vi "Teleop.vi"(10 "Match Info":T2={"Autonomous Elapsed Seconds"=0.0, "TeleOp Elapsed Seconds"=0.0, "Disabled Elapsed Seconds"=0.0, "Visited Autonomous"=FALSE, "Visited TeleOp"=FALSE, "Visited Disabled"=FALSE, "Autonomous Settings"={"Autonomous Style"=enum."Independent", "VI Refnum"=refnum}}, 11 "Call Context":T3) -> ()   [LabVIEW 2020]
doc: "This VI is called for each TeleOp packet received from the DS where the robot is not disabled. It is often used to read from the joysticks and update I/O or to update setpoints for timed control loops. It should complete and return within 20 milliseconds or it may miss DS packets."
uses:
  <vilib>/Rock Robotics/WPI/DriverStation/WPI_DriverStationDerivedRobotMode.ctl
  <vilib>/Rock Robotics/WPI/DriverStation/WPI_DriverStationMatch Info.ctl
  <vilib>/Rock Robotics/WPI/ThirdParty/Phoenix-LabVIEW/Motor Controller/Controls/CTRE_Phoenix_MotorControl_ControlMode.ctl
  <vilib>/Rock Robotics/WPI/Solenoid/WPI_SolenoidValue.ctl
  <vilib>/Rock Robotics/WPI/Utilities/WPI_GetSetVariantRefNum.vi
  <vilib>/Rock Robotics/Network Tables/NT Read Boolean.vi
  <vilib>/Rock Robotics/Network Tables/NT Read Number.vi
  <vilib>/Rock Robotics/Network Tables/NT Read String.vi
  <vilib>/Rock Robotics/Network Tables/NT Write Boolean.vi
  <vilib>/Rock Robotics/Network Tables/NT Write String.vi
  <vilib>/Rock Robotics/WPI/Solenoid/WPI_SolenoidSetEnum.vi
  <vilib>/Rock Robotics/WPI/ThirdParty/Phoenix-LabVIEW/Motor Controller/Get/CTRE_Phoenix_MotorController_IntegratedSensorData_TalonFX.vi
  <vilib>/Rock Robotics/Network Tables/NT Write Number.vi
  <vilib>/addons/control/pid/pid.llb/PID (DBL).vi
  <vilib>/addons/control/pid/NI_PID_pid.lvlib
panel:
  in  "PID gains 5":T1={"proportional gain (Kc)"=0.005, "integral time (Ti, min)"=0.0, "derivative time (Td, min)"=2e-05} {"derivative time (Td, min)" format="%.6f"; "integral time (Ti, min)" format="%.3f"; "proportional gain (Kc)" format="%.3f"}
  in  "Elevate want":dbl=-0.35
  in  "Intake want":dbl=0.75
  in  "Subtract rpm":dbl=2975.0
  out "% voltage":dbl
  out "voltage (V)":dbl
  out "Motor Volts":dbl
  out "rpm":dbl
  out "limelight tx":dbl
  out "limelight ty":dbl
  in  "Auto-Accept":bool
  in  "8togglePressed?":bool
  in  "Red/Blue":u32(colorbox)
  out "B":u8
  out "G":u8
  out "R":u8
  out "Color":u32(colorbox)
  out "Sample Slider 0":dbl(slide) scale=0.0..5.0
  out "Sample Boolean 1":bool
  out "Sample Boolean 0":bool
  # "-1"
  # "0"
  # ".75"
  # ".75"
  # "-.6"
  # "-.35"
  # ".1"
  # "1"
  # "-.1"
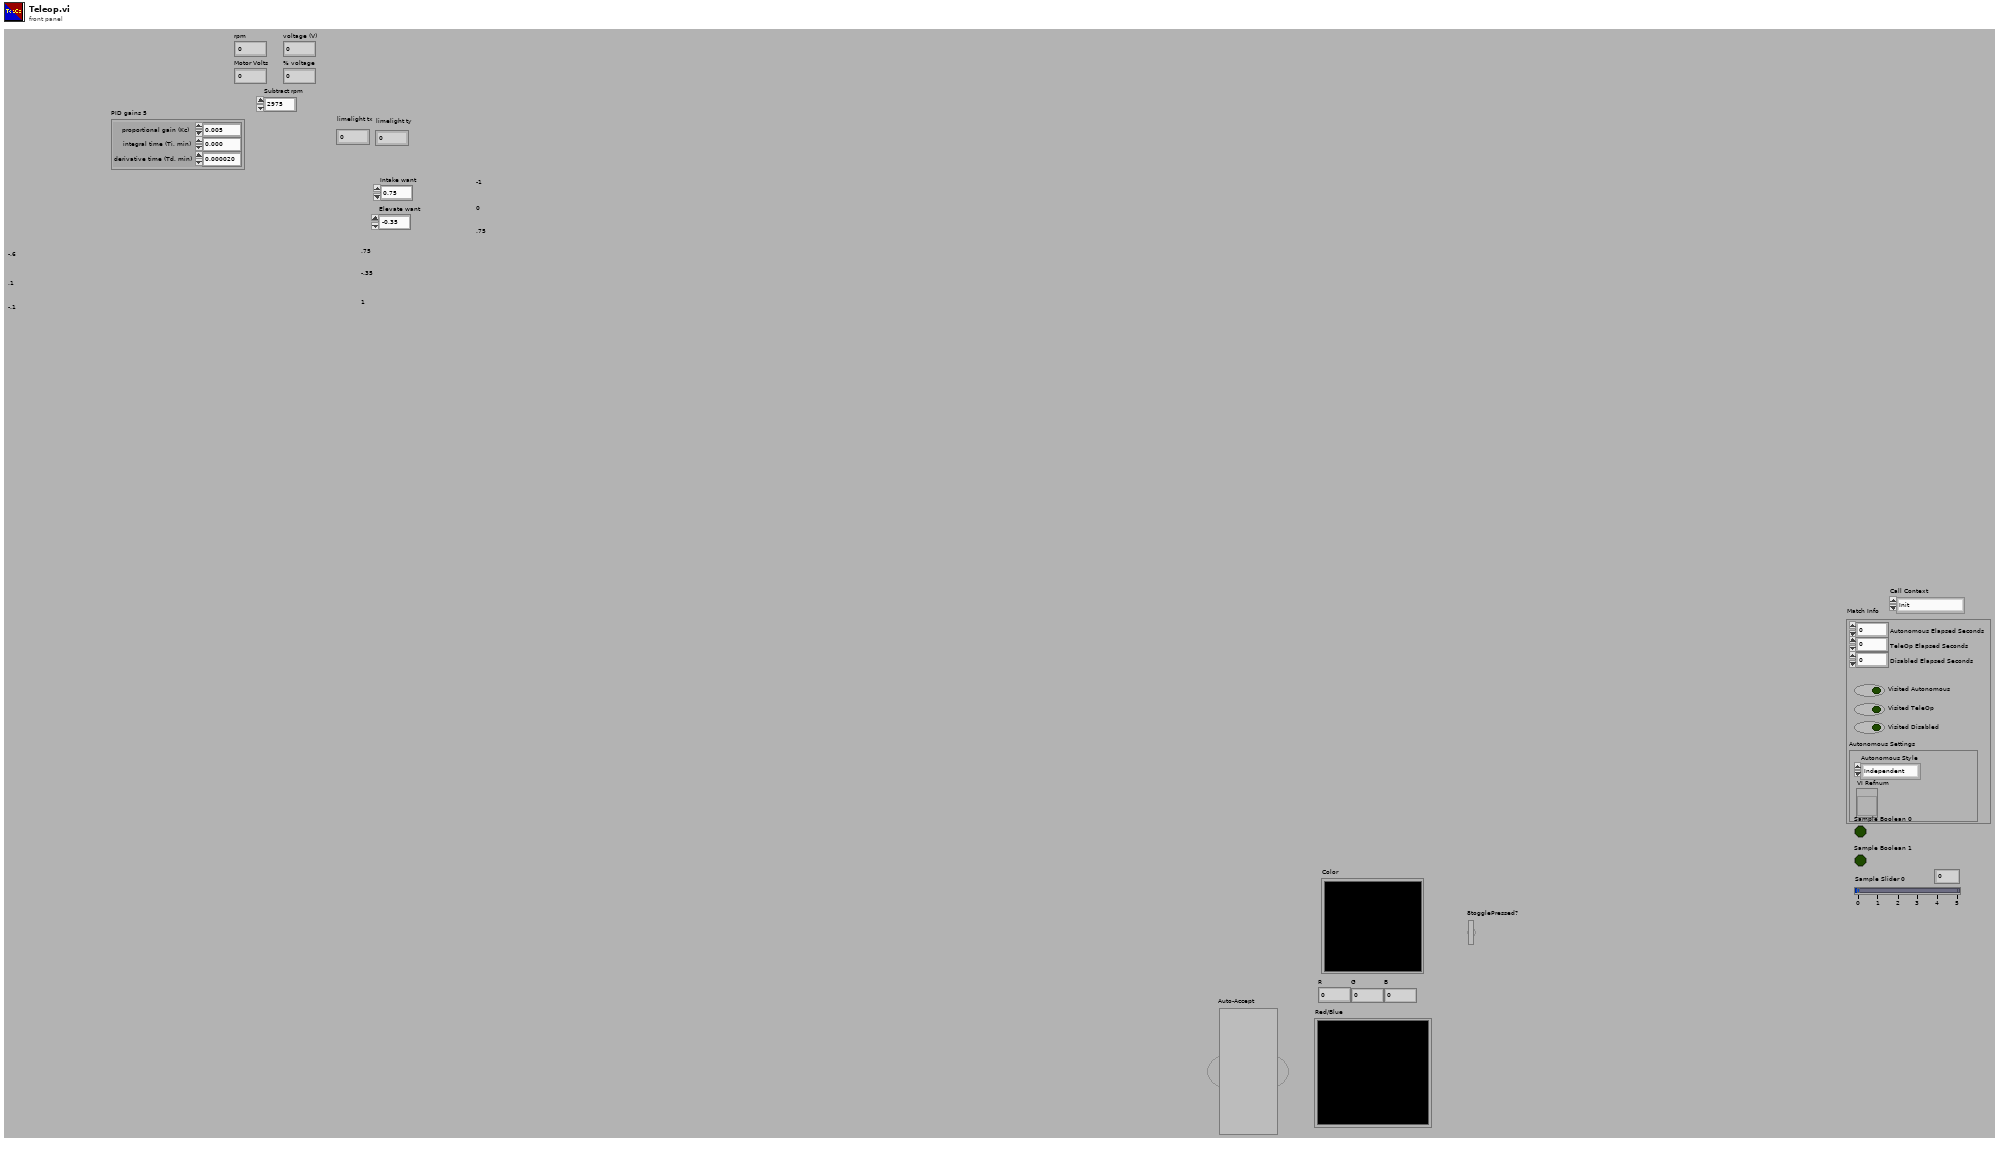
[diagram p1: front panel]
types:
  T1 = cluster{"proportional gain (Kc)":dbl, "integral time (Ti, min)":dbl, "derivative time (Td, min)":dbl}
  T2 = typedef "WPI_DriverStationMatch Info.ctl" = cluster{"Autonomous Elapsed Seconds":dbl, "TeleOp Elapsed Seconds":dbl, "Disabled Elapsed Seconds":dbl, "Visited Autonomous":bool, "Visited TeleOp":bool, "Visited Disabled":bool, "Autonomous Settings":cluster{"Autonomous Style":enum16{"Iterative", "Independent"}, "VI Refnum":refnum<vi>}}
  T3 = typedef "WPI_DriverStationDerivedRobotMode.ctl" = enum16{"Init", "Execute", "Stop"}
  T4 = typedef "CTRE_Phoenix_MotorControl_ControlMode.ctl" = u16
  T5 = typedef "WPI_SolenoidValue.ctl" = enum16{"Off", "On", "Forward", "Reverse"}
  T6 = typedef "WPI_MotorControlDeviceRef.ctl" = cluster{"DeviceStatus":errorcluster, "Type":T7, "PWM":cluster{"PWM Channel":T8, "DeadBand":T9}, "CAN":cluster{"Device Number":u8, "SetOutput VI Ref":variant, "GetOutput VI Ref":variant, "Enable VI Ref":variant, "Disable VI Ref":variant, "Data":variant}, "Invert":bool, "DIO PWM":cluster{"PWM \"Enable\" Channel":T8, "DIOChannel":T10, "PWM Rate":dbl}}
  T7 = typedef "WPI_MotorControlType.ctl" = enum16{"PWM", "CAN", "DIO PWM"}
  T8 = typedef "FPGA_DIOPWMChannel.ctl" = enum8{"PWM 0", "PWM 1", "PWM 2", "PWM 3", "PWM 4", "PWM 5", "PWM 6", "PWM 7", "PWM 8", "PWM 9", "PWM MXP 0", "PWM MXP 1", "PWM MXP 2", "PWM MXP 3", "PWM MXP 4", "PWM MXP 5", "PWM MXP 6", "PWM MXP 7", "PWM MXP 8", "PWM MXP 9", "Invalid"}
  T9 = typedef "WPI_PWMDeadband.ctl" = cluster{"Name":string, "maxPositivePwm":i32, "minPositivePwm":i32, "centerPwm":i32, "maxNegativePwm":i32, "minNegativePwm":i32, "angularRange":u16}
  T10 = typedef "FPGA_DIOChannel.ctl" = enum8{"DIO 0", "DIO 1", "DIO 2", "DIO 3", "DIO 4", "DIO 5", "DIO 6", "DIO 7", "DIO 8", "DIO 9", "DIO MXP 0", "DIO MXP 1", "DIO MXP 2", "DIO MXP 3", "DIO MXP 4", "DIO MXP 5", "DIO MXP 6", "DIO MXP 7", "DIO MXP 8", "DIO MXP 9", "DIO MXP 10", "DIO MXP 11", "DIO MXP 12", "DIO MXP 13", "DIO MXP 14", "DIO MXP 15", "SPI Port CS1", "SPI Port CS2", "SPI Port CS3", "SPI Port MISO", "SPI Port MOSI", "Invalid"}
  T11 = typedef "WPI_SolenoidDevRef.ctl" = cluster{"DevStatus":errorcluster, "Pneumatics Control Module":u8, "Forward Solenoid Channel":T12, "Reverse Solenoid Channel":T12}
  T12 = typedef "WPI_SolenoidChannel.ctl" = enum8{"Solenoid 0", "Solenoid 1", "Solenoid 2", "Solenoid 3", "Solenoid 4", "Solenoid 5", "Solenoid 6", "Solenoid 7", "Solenoid 8", "Solenoid 9", "Solenoid 10", "Solenoid 11", "Solenoid 12", "Solenoid 13", "Solenoid 14", "Solenoid 15", "Invalid"}
  T13 = typedef "WPI_CompressorDevRef.ctl" = cluster{"DevStatus":errorcluster, "Pneumatics Control Module":u8}
  T14 = typedef "WPI_SwitchDevRef.ctl" = cluster{"DevStatus":errorcluster, "DIO Channel":T10, "CntIndex":T15, "Normally Closed":bool}
  T15 = typedef "FPGA_CounterCtrSystemIndex.ctl" = enum8{"Ctr 0", "Ctr 1", "Ctr 2", "Ctr 3", "Ctr 4", "Ctr 5", "Ctr 6", "Ctr 7", "Invalid"}
  T16 = typedef "Color Sensor V3 DevRef.ctl" = cluster{"I2CDevRef":T17}
  T17 = typedef "WPI_I2CDevRef.ctl" = cluster{"DevStatus":errorcluster, "Device Address":u8, "Handle":i32, "I2C Bus":T18}
  T18 = typedef "i2c_bus.ctl" = enum16{"I2C On-Board", "I2C MXP", "Invalid"}
  T19 = typedef "WPI_JoystickDevRef.ctl" = cluster{"Device":T20}
  T20 = typedef "WPI_JoystickDeviceEnum.ctl" = enum16{"USB 0", "USB 1", "USB 2", "USB 3", "USB 4", "USB 5"}
  T21 = cluster{"A":bool, "B":bool, "X":bool, "Y":bool, "Left Bumper":bool, "Right Bumper":bool, "View Button":bool, "Menu Button":bool, "Left Joystick Press":bool, "Right Joystick Press":bool, "Left Thumbpad X Axis":dbl, "Left Thumbpad Y Axis":dbl, "Left Trigger":dbl, "Right Trigger":dbl, "Right Thumbpad X Axis":dbl, "Right Thumbpad Y Axis":dbl, "Driver - Trigger":bool, "Driver - Middle Thumb":bool, "Driver - Left Thumb":bool, "Driver - Right Thumb":bool, "Driver - Left Top Left ":bool, "Driver - Left Top Middle":bool, "Driver - Left Top Right":bool, "Driver - Left Bottom Right":bool, "Driver - Left Bottom Middle":bool, "Driver - Left Bottom Left":bool, "Driver - Right Top Right":bool, "Driver - Right Top Middle":bool, "Driver - Right Top Left":bool, "Driver - Right Bottom Left":bool, "Driver - Right Bottom Middle":bool, "Driver - Right Bottom Right":bool, "Driver - X Axis":dbl, "Driver - Y Axis":dbl, "Driver - Z Axis":dbl}
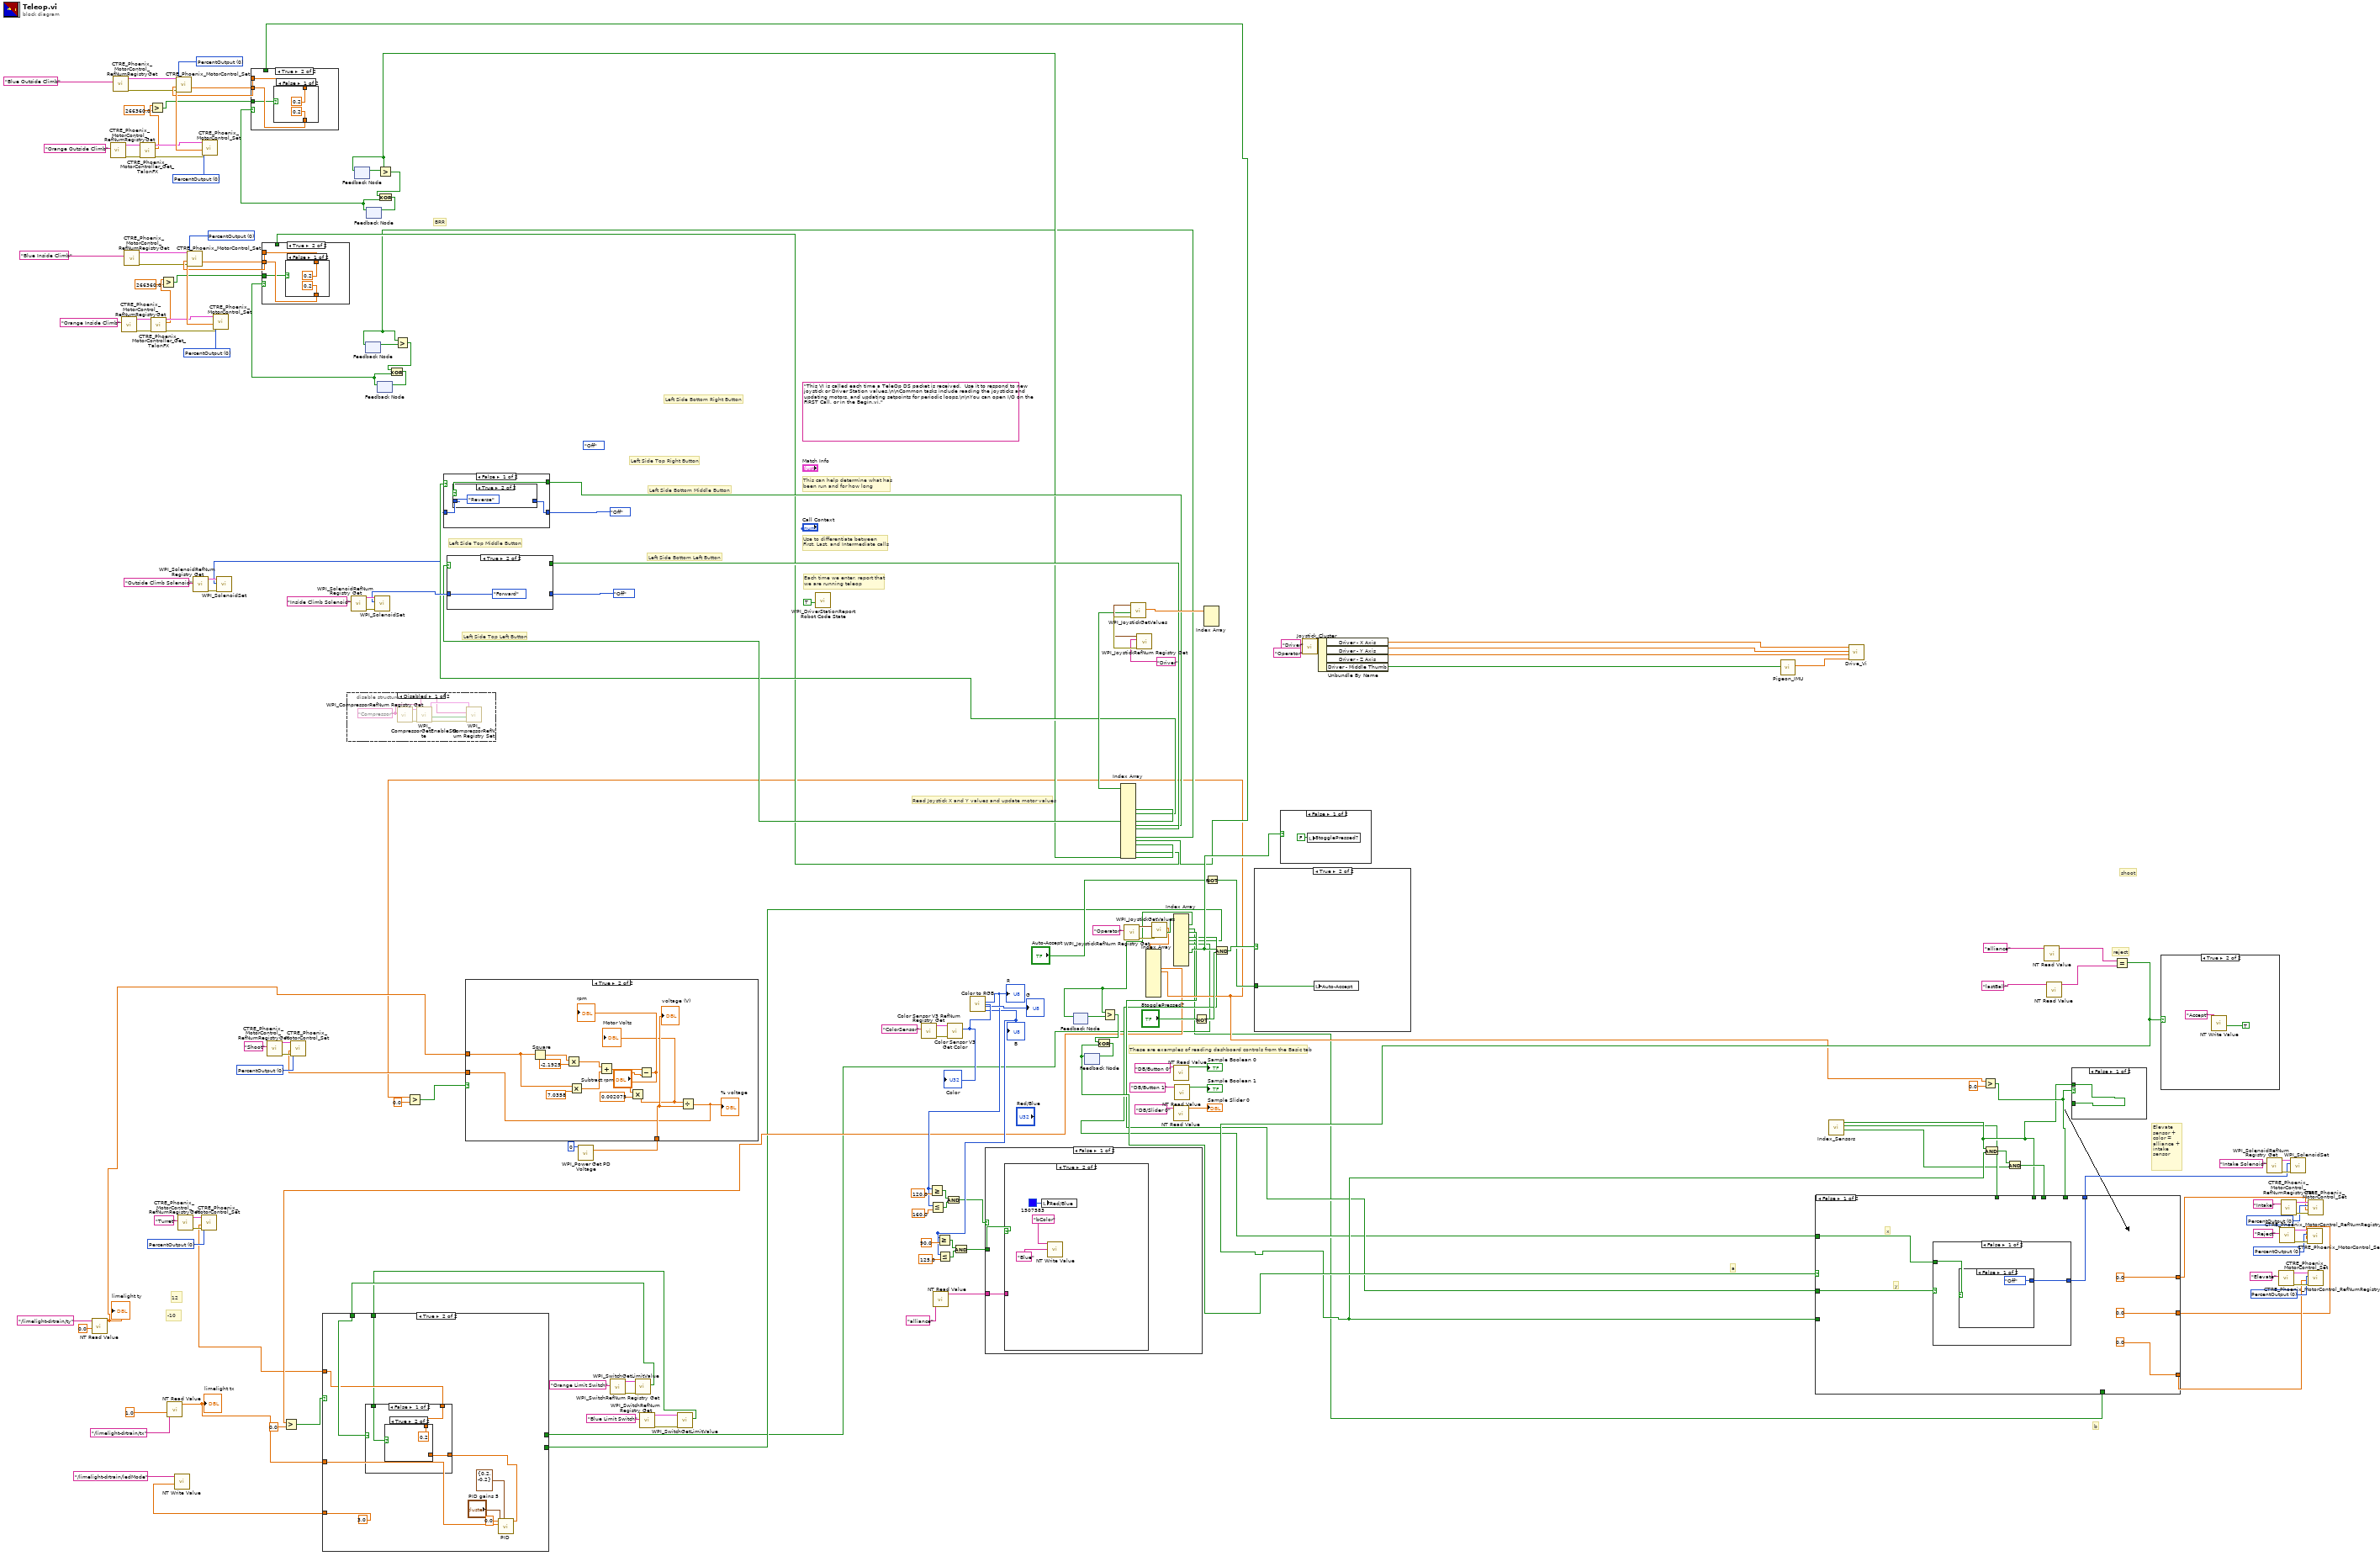
[diagram p0: block diagram]
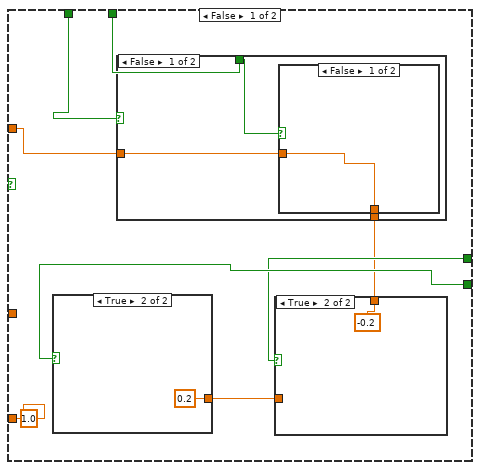
[diagram p2: hidden frame]
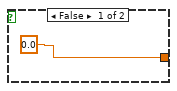
[diagram p4: hidden frame]
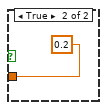
[diagram p5: hidden frame]
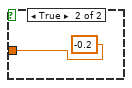
[diagram p6: hidden frame]
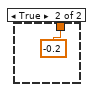
[diagram p8: hidden frame]
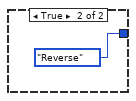
[diagram p9: hidden frame]
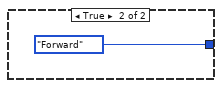
[diagram p10: hidden frame]
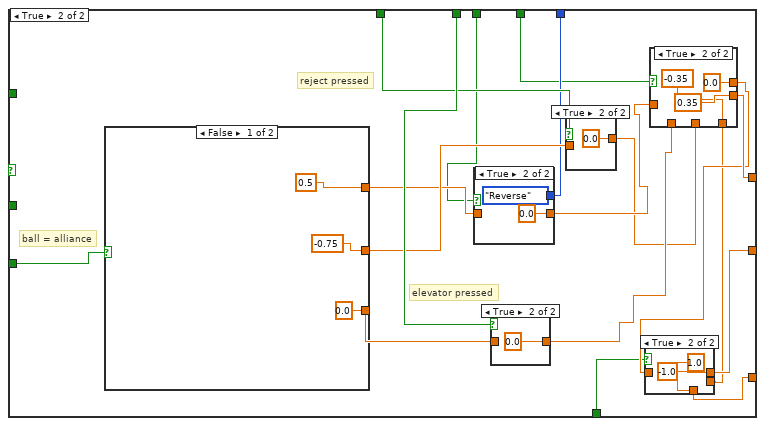
[diagram p11: hidden frame]
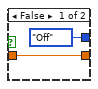
[diagram p14: hidden frame]
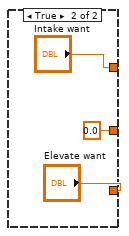
[diagram p17: hidden frame]
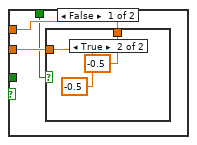
[diagram p18: hidden frame]
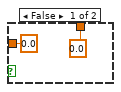
[diagram p19: hidden frame]
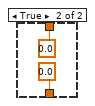
[diagram p20: hidden frame]
diagram:
  w59 = T4 0 items=["PercentOutput"=0, "Position"=1, "Velocity"=2, "Current"=3, "Follower"=5, "MotionProfile"=6, "MotionMagic"=7, "MotionProfileArc"=10, "Disabled"=15] ("Control Mode")
  w60 = T4 0 items=["PercentOutput"=0, "Position"=1, "Velocity"=2, "Current"=3, "Follower"=5, "MotionProfile"=6, "MotionMagic"=7, "MotionProfileArc"=10, "Disabled"=15] ("Control Mode")
  (unwired) WPI_SolenoidValue."Off" ("inside climb start")
  w78 = T4 0 items=["PercentOutput"=0, "Position"=1, "Velocity"=2, "Current"=3, "Follower"=5, "MotionProfile"=6, "MotionMagic"=7, "MotionProfileArc"=10, "Disabled"=15] ("Control Mode")
  w79 = T4 0 items=["PercentOutput"=0, "Position"=1, "Velocity"=2, "Current"=3, "Follower"=5, "MotionProfile"=6, "MotionMagic"=7, "MotionProfileArc"=10, "Disabled"=15] ("Control Mode")
  w112 = T4 0 items=["PercentOutput"=0, "Position"=1, "Velocity"=2, "Current"=3, "Follower"=5, "MotionProfile"=6, "MotionMagic"=7, "MotionProfileArc"=10, "Disabled"=15] ("Control Mode")
  w120 = T4 0 items=["PercentOutput"=0, "Position"=1, "Velocity"=2, "Current"=3, "Follower"=5, "MotionProfile"=6, "MotionMagic"=7, "MotionProfileArc"=10, "Disabled"=15] ("Control Mode")
  w131 = T4 0 items=["PercentOutput"=0, "Position"=1, "Velocity"=2, "Current"=3, "Follower"=5, "MotionProfile"=6, "MotionMagic"=7, "MotionProfileArc"=10, "Disabled"=15] ("Control Mode")
  w132 = T4 0 items=["PercentOutput"=0, "Position"=1, "Velocity"=2, "Current"=3, "Follower"=5, "MotionProfile"=6, "MotionMagic"=7, "MotionProfileArc"=10, "Disabled"=15] ("Control Mode")
  w133 = T4 0 items=["PercentOutput"=0, "Position"=1, "Velocity"=2, "Current"=3, "Follower"=5, "MotionProfile"=6, "MotionMagic"=7, "MotionProfileArc"=10, "Disabled"=15] ("Control Mode")
  (unwired) "This VI is called each time a TeleOp DS packet is received.  Use it to respond to new joystick or Driver Station values.\n\nCommon tasks include reading the joysticks and updating motors, and updating setpoints for periodic loops.\n\nYou can open I/O on the FIRST Call, or in the Begin.vi."
  # "Elevate sensor + color = alliance + intake sensor"
  # "b"
  # "a"
  # "BRR"
  # "Left Side Bottom Right Button"
  # "Left Side Top Right Button"
  # "Left Side Bottom Middle Button"
  # "Left Side Top Middle Button"
  # "Left Side Bottom Left Button"
  # "Left Side Top Left Button"
  # "shoot"
  # "reject"
  # "12"
  # "-10"
  # "These are examples of reading dashboard controls from the Basic tab"
  # "Read Joystick X and Y values and update motor values"
  # "Each time we enter, report that\nwe are running teleop"
  # "Use to differentiate between\nFirst, Last, and Intermediate calls"
  # "This can help determine what has\nbeen run and for how long"
  n1 = call-poly <vilib>:"NT Read Value.vi"("Default Value"=0.0, "Name"="/limelight-drtrain/ty") -> ("Numeric"=w90:dbl)  [unwired: 8 in, 1 out]
  "limelight ty" <- w90
  n2 = call <vilib>:"CTRE_Phoenix_MotorControl_RefNumRegistryGet.vi"("refnum name"="Orange Outside Climb") -> ("error out"=w56:errorcluster, "PhoenixMotorControlDevRef"=w55:T6)  [unwired: 9 in]
  n3 = call <vilib>:"CTRE_Phoenix_MotorControl_RefNumRegistryGet.vi"("refnum name"="Blue Outside Climb") -> ("error out"=w51:errorcluster, "PhoenixMotorControlDevRef"=w52:T6)  [unwired: 9 in]
  n4 = call <vilib>:"CTRE_Phoenix_MotorControl_RefNumRegistryGet.vi"("refnum name"="Orange Inside Climb") -> ("error out"=w75:errorcluster, "PhoenixMotorControlDevRef"=w74:T6)  [unwired: 9 in]
  n5 = call <vilib>:"CTRE_Phoenix_MotorControl_RefNumRegistryGet.vi"("refnum name"="Blue Inside Climb") -> ("error out"=w70:errorcluster, "PhoenixMotorControlDevRef"=w71:T6)  [unwired: 9 in]
  n6 = call-poly <vilib>:"CTRE_Phoenix_MotorController_Get_TalonFX.vi"("PhoenixMotorControlDevRef"=w55, "error in"=w56) -> ("PhoenixMotorControlDevRef"=w54:T6, "Position"=w46:dbl, "error out"=w53:errorcluster)  [unwired: 9 in, 2 out]
  n7 = Greater?(x=w46, y=266360.0) -> (0:w44:bool)
  n8 = call-poly <vilib>:"CTRE_Phoenix_MotorController_Get_TalonFX.vi"("PhoenixMotorControlDevRef"=w74, "error in"=w75) -> ("PhoenixMotorControlDevRef"=w73:T6, "Position"=w65:dbl, "error out"=w72:errorcluster)  [unwired: 9 in, 2 out]
  n9 = Greater?(x=w65, y=266360.0) -> (0:w63:bool)
  n10 = call-poly <vilib>:"NT Read Value.vi"("Default Value"=1.0, "Name"="/limelight-drtrain/tx") -> ("Numeric"=w20:dbl)  [unwired: 8 in, 1 out]
  "limelight tx" <- w20
  n11 = call <vilib>:"CTRE_Phoenix_MotorControl_RefNumRegistryGet.vi"("refnum name"="Turret") -> ("error out"=w115:errorcluster, "PhoenixMotorControlDevRef"=w114:T6)  [unwired: 9 in]
  n12 = call <vilib>:"WPI_SolenoidRefNum Registry Get.vi"("refnum name"="Outside Climb Solenoid") -> ("error out"=w107:errorcluster, "SolenoidDevRef"=w106:T11)  [unwired: 9 in]
  n13 = call <vilib>:"CTRE_Phoenix_MotorControl_RefNumRegistryGet.vi"("refnum name"="Shoot") -> ("error out"=w123:errorcluster, "PhoenixMotorControlDevRef"=w122:T6)  [unwired: 9 in]
  n14 = disable-structure shown="Disabled" {
    frame Disabled {
      w182 = "Compressor" ("refnum name")
      n15 = call <vilib>:"WPI_CompressorRefNum Registry Get.vi"("refnum name"=w182) -> ("error out"=w187:errorcluster, "CompressorDevRef"=w186:T13)  [unwired: 9 in]
      n16 = call <vilib>:"WPI_CompressorGetEnableState.vi"("error in (no error)"=w187, "CompressorDevRef"=w186) -> ("error out"=w185:errorcluster, "Compressor Running"=w184:bool, "CompressorDevRef"=w183:T13)  [unwired: 3 in, 4 out]
      n17 = call <vilib>:"WPI_CompressorRefNum Registry Set.vi"("error in (no error)"=w185, "Test Mode Only"=w184, "refnum name"=w182, "CompressorDevRef"=w183) -> ()  [unwired: 6 in, 2 out]
    }
    frame Enabled {
    }
  }
  n18 = call <vilib>:"WPI_SolenoidRefNum Registry Get.vi"("refnum name"="Inside Climb Solenoid") -> ("error out"=w104:errorcluster, "SolenoidDevRef"=w103:T11)  [unwired: 9 in]
  n19 = feedback #1() -> (w50:bool)  [unwired: 1 in]
  n20 = feedback #2() -> (w69:bool)  [unwired: 1 in]
  n21 = feedback #3() -> (w47:bool)  [unwired: 1 in]
  n22 = feedback #4() -> (w66:bool)  [unwired: 1 in]
  n23 = call <vilib>:"WPI_Power Get PD Voltage.vi"("Power Distribution Panel (def)"=u8 0) -> ("voltage (V)"=w91:dbl)  [unwired: 13 in, 1 out]
  n24 = call <vilib>:"WPI_SwitchRefNum Registry Get.vi"("refnum name"="Orange Limit Switch") -> ("error out"=w98:errorcluster, "SwitchDevRef"=w97:T14)  [unwired: 9 in]
  n25 = call <vilib>:"WPI_SwitchGetLimitValue.vi"("error in (no error)"=w98, "SwitchDevRef"=w97) -> ("Switch Pressed"=w18:bool)  [unwired: 7 in, 2 out]
  n26 = call <vilib>:"WPI_SwitchRefNum Registry Get.vi"("refnum name"="Blue Limit Switch") -> ("error out"=w95:errorcluster, "SwitchDevRef"=w94:T14)  [unwired: 9 in]
  n27 = call <vilib>:"WPI_SwitchGetLimitValue.vi"("error in (no error)"=w95, "SwitchDevRef"=w94) -> ("Switch Pressed"=w17:bool)  [unwired: 7 in, 2 out]
  n28 = call <vilib>:"WPI_DriverStationReport Robot Code State.vi"("TeleOp"=TRUE ("Autonomous")) -> ()  [unwired: 10 in, 1 out]
  n29 = call <vilib>:"Color Sensor V3 RefNum Registry Get.vi"("refnum name"="ColorSensor") -> ("error out"=w167:errorcluster, "ColorSensorDevRef"=w168:T16)  [unwired: 9 in]
  n30 = call-poly <vilib>:"NT Read Value.vi"("Name"="alliance") -> ("String"=w117:string)  [unwired: 9 in, 1 out]
  n31 = call <vilib>:"Color Sensor V3 Get Color.vi"("error in (no error)"=w167, "ColorSensorDevRef"=w168) -> ("Color"=w166:u32)  [unwired: 6 in, 3 out]
  "Color" <- w166
  n32 = call <vilib>:"Color to RGB.vi"("Color"=w166) -> ("R"=w160:u8, "G"=→"G":u8, "B"=w155:u8)  [unwired: 1 out]
  "R" <- w160
  "B" <- w155
  n33 = Greater Or Equal?(x=w160, y=120.0) -> (x >= y?=w163:bool)
  n34 = Less Or Equal?(x=w160, y=160.0) -> (x <= y?=w164:bool)
  n35 = Greater Or Equal?(x=w155, y=90.0) -> (x >= y?=w158:bool)
  n36 = Less Or Equal?(x=w155, y=125.0) -> (x <= y?=w159:bool)
  n37 = And(x=w163, y=w164) -> (x .and. y?=w144:bool)
  n38 = And(x=w158, y=w159) -> (x .and. y?=w143:bool)
  n39 = case shown="False" w144 {
    tunnel: w143 -> [w189 _]
    tunnel: w117 -> [w188 _]
    frame False {
      n40 = case shown="True" w189 {
        tunnel: w188 -> [w190 _]
        frame False {
          n41 = disable-structure shown="Disabled" {
            disable-tunnel: w190 -> [w191 _]
            frame Disabled {
              n42 = case shown="\"Blue\", Default" w191 {
                frame "Blue", Default {
                  n43 = call-poly <vilib>:"NT Write Value.vi"("String"="Red", "Name"="bColor") -> ()  [unwired: 9 in, 1 out]
                  n44 = local write "Red/Blue"(u32 16711680 ("Color Box")) -> ()
                }
                frame "Red" {
                  n45 = local write "Red/Blue"(u32 16860 ("Red/Blue")) -> ()
                  n46 = call-poly <vilib>:"NT Write Value.vi"("String"="Blue", "Name"="bColor") -> ()  [unwired: 9 in, 1 out]
                }
              }
            }
            frame Enabled {
            }
          }
        }
        frame True {
          n47 = local write "Red/Blue"(u32 1507583 ("Color Box")) -> ()
          n48 = call-poly <vilib>:"NT Write Value.vi"("String"="Blue", "Name"="bColor") -> ()  [unwired: 9 in, 1 out]
        }
      }
    }
    frame True {
      n49 = call-poly <vilib>:"NT Write Value.vi"("String"="Red", "Name"="bColor") -> ()  [unwired: 9 in, 1 out]
      n50 = local write "Red/Blue"(u32 16714752) -> ()
    }
  }
  n51 = feedback #5() -> (w127:bool)  [unwired: 1 in]
  n52 = feedback #6() -> (w43:bool)  [unwired: 1 in]
  n53 = call <vilib>:"WPI_JoystickRefNum Registry Get.vi"("refnum name"="Operator") -> ("error out"=w153:errorcluster, "JoystickDevRef"=w152:T19)  [unwired: 9 in]
  n54 = call <vilib>:"WPI_JoystickRefNum Registry Get.vi"("refnum name"="Driver") -> ("error out"=w180:errorcluster, "JoystickDevRef"=w179:T19)  [unwired: 9 in]
  n55 = call <vilib>:"WPI_JoystickGetValues.vi"("error in (no error)"=w180, "JoystickDevRef"=w179) -> ("Buttons"=w176:bool[], "Axes"=w177:dbl[])  [unwired: 5 in, 3 out]
  n56 = Index Array(array=w176) -> (element #5=w86:bool, element #6=w84:bool, element #9=w83:bool, element #10=w87:bool, element #12=w32:bool, element #13=w35:bool, element #14=w34:bool, element #16=w33:bool)  [unwired: 17 in, 9 out]
  n57 = case shown="True" w47 {
    tunnel: [w205 w212] -> w58
    tunnel: [w206 w213] -> w57
    tunnel: w35 -> [w204 _]
    tunnel: w44 -> [_ w211]
    frame False {
      n58 = case shown="True" w204 {
        tunnel: [0.0 ("Output") -0.5 ("Output")] -> w206
        tunnel: [0.0 ("Output") -0.5 ("Output")] -> w205
        frame False {
        }
        frame True {
        }
      }
    }
    frame True {
      n59 = case shown="False" w211 {
        tunnel: [0.2 ("Output") 0.0 ("Output")] -> w213
        tunnel: [0.2 ("Output") 0.0 ("Output")] -> w212
        frame False {
        }
        frame True {
        }
      }
    }
  }
  n60 = call <vilib>:"CTRE_Phoenix_MotorControl_Set.vi"("error in (no error)"=w51, "Output"=w57, "Control Mode"=w60, "PhoenixMotorControlDevRef"=w52) -> ()  [unwired: 6 in, 2 out]
  n61 = call <vilib>:"CTRE_Phoenix_MotorControl_Set.vi"("error in (no error)"=w53, "Output"=w58, "Control Mode"=w59, "PhoenixMotorControlDevRef"=w54) -> ()  [unwired: 6 in, 2 out]
  n62 = case shown="True" w66 {
    tunnel: [w219 w226] -> w77
    tunnel: [w220 w227] -> w76
    tunnel: w33 -> [w218 _]
    tunnel: w63 -> [_ w225]
    frame False {
      n63 = case shown="False" w218 {
        tunnel: [0.0 ("Output") -0.5 ("Output")] -> w220
        tunnel: [0.0 ("Output") -0.5 ("Output")] -> w219
        frame False {
        }
        frame True {
        }
      }
    }
    frame True {
      n64 = case shown="False" w225 {
        tunnel: [0.2 ("Output") 0.0 ("Output")] -> w227
        tunnel: [0.2 ("Output") 0.0 ("Output")] -> w226
        frame False {
        }
        frame True {
        }
      }
    }
  }
  n65 = call <vilib>:"CTRE_Phoenix_MotorControl_Set.vi"("error in (no error)"=w70, "Output"=w76, "Control Mode"=w79, "PhoenixMotorControlDevRef"=w71) -> ()  [unwired: 6 in, 2 out]
  n66 = call <vilib>:"CTRE_Phoenix_MotorControl_Set.vi"("error in (no error)"=w72, "Output"=w77, "Control Mode"=w78, "PhoenixMotorControlDevRef"=w73) -> ()  [unwired: 6 in, 2 out]
  n67 = feedback-in #1(w34) -> ()
  n68 = feedback-in #2(w32) -> ()
  n69 = Greater?(x=w34, y=w50) -> (0:w49:bool)
  n70 = Exclusive Or(1:w47, 2:w49) -> (0:w48:bool)
  n71 = feedback-in #3(w48) -> ()
  n72 = Greater?(x=w32, y=w69) -> (0:w68:bool)
  n73 = Exclusive Or(1:w66, 2:w68) -> (0:w67:bool)
  n74 = feedback-in #4(w67) -> ()
  n75 = case shown="False" w84 {
    tunnel: [w232 WPI_SolenoidValue."Forward" ("inside climb start")] -> w82
    tunnel: WPI_SolenoidValue."Off" ("inside climb start") -> [w233 _]
    tunnel: w83 -> [w234 _]
    frame False {
      n76 = case shown="True" w234 {
        tunnel: w233 -> [w235 _]
        tunnel: [w235 WPI_SolenoidValue."Reverse" ("inside climb start")] -> w232
        frame False {
        }
        frame True {
        }
      }
    }
    frame True {
    }
  }
  n77 = call-poly <vilib>:"WPI_SolenoidSet.vi"("error in (no error)"=w107, "Value"=w82, "SolenoidDevRef"=w106) -> ()  [unwired: 7 in, 2 out]
  n78 = case shown="True" w86 {
    tunnel: [w238 WPI_SolenoidValue."Forward" ("inside climb start")] -> w89
    tunnel: WPI_SolenoidValue."Off" ("inside climb start") -> [w239 _]
    tunnel: w87 -> [w240 _]
    frame False {
      n79 = case shown="False" w240 {
        tunnel: w239 -> [w241 _]
        tunnel: [w241 WPI_SolenoidValue."Reverse" ("inside climb start")] -> w238
        frame False {
        }
        frame True {
        }
      }
    }
    frame True {
    }
  }
  n80 = call-poly <vilib>:"WPI_SolenoidSet.vi"("error in (no error)"=w104, "Value"=w89, "SolenoidDevRef"=w103) -> ()  [unwired: 7 in, 2 out]
  n81 = call <vilib>:"WPI_JoystickGetValues.vi"("error in (no error)"=w153, "JoystickDevRef"=w152) -> ("Buttons"=w151:bool[], "Axes"=w31:dbl[])  [unwired: 5 in, 3 out]
  n82 = Index Array(array=w31) -> (element #3=w21:dbl, element #4=w26:dbl)  [unwired: 10 in, 8 out]
  n83 = Greater?(x=w21, y=0.0) -> (0:w22:bool)
  n84 = Greater?(x=w26, y=0.0) -> (0:w27:bool)
  n85 = case shown="True" w27 {
    tunnel: [0.0 ("Shoot %") w246] -> w119
    tunnel: w90 -> [_ w254]
    tunnel: w91 -> [_ w248]
    frame False {
    }
    frame True {
      n86 = Square(x=w254) -> (x^2=w257:dbl)
      n87 = Multiply(x=w257, y=-2.1925) -> (x*y=w255:dbl)
      n88 = Multiply(x=w254, y=7.0358) -> (x*y=w252:dbl)
      n89 = Add(x=w255, y=w252) -> (x+y=w251:dbl)
      n90 = Subtract(x=w251, y="Subtract rpm") -> (x-y=w250:dbl)
      "rpm" <- w250
      n91 = Multiply(x=w250, y=0.002075) -> (x*y=w247:dbl)
      "Motor Volts" <- w247
      n92 = Divide(x=w247, y=w248) -> (x/y=w246:dbl)
      "% voltage" <- w246
      "voltage (V)" <- w248
    }
  }
  n93 = call <vilib>:"CTRE_Phoenix_MotorControl_Set.vi"("error in (no error)"=w123, "Output"=w119, "Control Mode"=w120, "PhoenixMotorControlDevRef"=w122) -> ()  [unwired: 6 in, 2 out]
  n94 = Index Array(array=w151) -> (element #1=w126:bool, element #2=w1:bool, element #3=w25:bool, element #4=w24:bool, element #5=w16:bool, element #6=w15:bool, element #8=w146:bool)  [unwired: 11 in, 4 out]
  n95 = case shown="True" w22 {
    tunnel: w20 -> [_ w284]
    tunnel: [w259 w279] -> w19
    tunnel: w18 -> [w265 w280]
    tunnel: w17 -> [w264 w277]
    tunnel: w16 -> [w263 _]
    tunnel: w15 -> [w262 _]
    tunnel: [1.0 ("Numeric") 3.0 ("Numeric")] -> w13
    frame False {
      n96 = case shown="True" w263 {
        tunnel: [0.0 ("output") 0.2 ("output")] -> w261
        frame False {
        }
        frame True {
        }
      }
      n97 = case shown="True" w262 {
        tunnel: w261 -> [w266 _]
        tunnel: [w266 -0.2 ("output")] -> w260
        frame False {
        }
        frame True {
        }
      }
      n98 = case shown="False" w265 {
        tunnel: w264 -> [w272 _]
        tunnel: w260 -> [w271 _]
        tunnel: [w270 -0.2 ("output")] -> w259
        frame False {
          n99 = case shown="False" w272 {
            tunnel: w271 -> [w273 _]
            tunnel: [w273 0.2 ("output")] -> w270
            frame False {
            }
            frame True {
            }
          }
        }
        frame True {
        }
      }
    }
    frame True {
      n100 = call-poly <vilib>:"PID.vi"("output range"=cluster{"output high":dbl, "output low":dbl} {"output high"=0.2, "output low"=-0.2}, "PID gains"="PID gains 5", "process variable"=w284, "setpoint"=0.0) -> ("output"=w278:dbl)  [unwired: 6 in, 1 out]
      n101 = case shown="False" w280 {
        tunnel: [w286 -0.2 ("output")] -> w279
        tunnel: w278 -> [w285 _]
        tunnel: w277 -> [w287 _]
        frame False {
          n102 = case shown="True" w287 {
            tunnel: [w288 0.2 ("output")] -> w286
            tunnel: w285 -> [w288 _]
            frame False {
            }
            frame True {
            }
          }
        }
        frame True {
        }
      }
    }
  }
  n103 = call-poly <vilib>:"NT Write Value.vi"("Numeric"=w13, "Name"="/limelight-drtrain/ledMode") -> ()  [unwired: 9 in, 1 out]
  n104 = call <vilib>:"CTRE_Phoenix_MotorControl_Set.vi"("error in (no error)"=w115, "Output"=w19, "Control Mode"=w112, "PhoenixMotorControlDevRef"=w114) -> ()  [unwired: 6 in, 2 out]
  n105 = feedback-in #5(w126) -> ()
  n106 = Greater?(x=w126, y=w127) -> (0:w125:bool)
  n107 = Exclusive Or(1:w43, 2:w125) -> (0:w124:bool)
  n108 = feedback-in #6(w124) -> ()
  n109 = call-poly <vilib>:"NT Read Value.vi"("Name"="DB/Button 0" ("refnum name")) -> ("Boolean"=→"Sample Boolean 0":bool)  [unwired: 9 in, 1 out]
  n110 = call-poly <vilib>:"NT Read Value.vi"("Name"="DB/Slider 0" ("refnum name")) -> ("Numeric"=→"Sample Slider 0":dbl)  [unwired: 9 in, 1 out]
  n111 = call-poly <vilib>:"NT Read Value.vi"("Name"="DB/Button 1" ("refnum name")) -> ("Boolean"=→"Sample Boolean 1":bool)  [unwired: 9 in, 1 out]
  n112 = Not(x="8togglePressed?") -> (.not. x?=w149:bool)
  n113 = Index Array(array=w177) -> ()  [unwired: 3 in, 3 out]
  n114 = Not(x="Auto-Accept") -> (.not. x?=w147:bool)
  n115 = And(x=w146, y=w149) -> (x .and. y?=w148:bool)
  n116 = case shown="True" w148 {
    tunnel: w147 -> [_ w291]
    frame False {
    }
    frame True {
      n117 = local write "Auto-Accept"(w291) -> ()
    }
  }
  n118 = case shown="False" w146 {
    frame False {
      n119 = local write "8togglePressed?"(FALSE ("togglePressed?")) -> ()
    }
    frame True {
      n120 = local write "8togglePressed?"(TRUE ("togglePressed?")) -> ()
    }
  }
  n121 = call "Joystick_Cluster.vi"("Xbox"="Operator", "Thrustmaster"="Driver") -> ("Joystick Output"=w10:T21)  [unwired: 9 in]
  n122 = Unbundle By Name(w10) -> ("Driver - X Axis"=w9:dbl, "Driver - Y Axis"=w8:dbl, "Driver - Z Axis"=w7:dbl, "Driver - Middle Thumb"=w6:bool)
  n123 = call "Pigeon_IMU.vi"("T/F"=w6) -> ("Yaw"=w5:dbl)  [unwired: 10 in]
  n124 = call "Index_Sensors.vi"() -> ("Intake Pressed"=w2:bool, "Reject Pressed"=w3:bool, "Elevate Pressed"=w4:bool)  [unwired: 9 in]
  n125 = call "Drive_Vi.vi"("Yaw"=w5, "Z"=w7, "Y"=w8, "X"=w9) -> ()  [unwired: 8 in]
  n126 = Greater?(x=w26, y=0.0) -> (0:w29:bool)
  n127 = call-poly <vilib>:"NT Read Value.vi"("Name"="alliance") -> ("String"=w130:string)  [unwired: 9 in, 1 out]
  n128 = call-poly <vilib>:"NT Read Value.vi"("Name"="lastBall") -> ("String"=w116:string)  [unwired: 9 in, 1 out]
  n129 = case shown="False" w29 {
    tunnel: w4 -> [w294 _]
    tunnel: [w294 FALSE ("Switch Pressed")] -> _
    frame False {
    }
    frame True {
    }
  }
  n130 = Equal?(x=w130, y=w116) -> (x = y?=w38:bool)
  n131 = And(x=w4, y=w38) -> (x .and. y?=w39:bool)
  n132 = And(x=w39, y=w2) -> (x .and. y?=w37:bool)
  n133 = case shown="False" w43 {
    tunnel: w38 -> [_ w324]
    tunnel: [0.0 ("Intake want") w316] -> w41
    tunnel: [0.0 ("Elevate 1") w308] -> w42
    tunnel: w4 -> [_ w323]
    tunnel: [0.0 ("Reject no want") w311] -> w40
    tunnel: w3 -> [_ w321]
    tunnel: w37 -> [_ w307]
    tunnel: [w298 w318] -> w36
    tunnel: w29 -> [_ w314]
    tunnel: w1 -> [_ w310]
    tunnel: w25 -> [w297 _]
    tunnel: w24 -> [w296 _]
    frame False {
      # "x"
      # "y"
      n134 = case shown="False" w297 {
        tunnel: [w303 WPI_SolenoidValue."Forward" ("Value")] -> w298
        tunnel: w296 -> [w302 _]
        frame False {
          n135 = case shown="False" w302 {
            tunnel: [WPI_SolenoidValue."Off" ("Value") WPI_SolenoidValue."Reverse" ("Value")] -> w303
            frame False {
            }
            frame True {
            }
          }
        }
        frame True {
        }
      }
    }
    frame True {
      # "reject pressed"
      # "elevator pressed"
      # "ball = alliance"
      n136 = case shown="False" w324 {
        tunnel: [0.0 ("Elevate want") "Elevate want"] -> w322
        tunnel: [0.5 ("Intake 1") "Intake want"] -> w319
        tunnel: [-0.75 ("Reject no want") 0.0 ("Reject no want")] -> w320
        frame False {
        }
        frame True {
        }
      }
      n137 = case shown="True" w307 {
        tunnel: w319 -> [w336 _]
        tunnel: [w336 0.0 ("Intake want")] -> w317
        tunnel: [WPI_SolenoidValue."Off" ("Value") WPI_SolenoidValue."Reverse" ("Value")] -> w318
        frame False {
        }
        frame True {
        }
      }
      n138 = case shown="True" w323 {
        tunnel: [w341 0.0 ("Elevate 1")] -> w315
        tunnel: w322 -> [w341 _]
        frame False {
        }
        frame True {
        }
      }
      n139 = case shown="True" w321 {
        tunnel: w320 -> [w339 _]
        tunnel: [w339 0.0 ("Reject no want")] -> w313
        frame False {
        }
        frame True {
        }
      }
      n140 = case shown="True" w314 {
        tunnel: w317 -> [w331 _]
        tunnel: [w331 0.35 ("Intake want")] -> w316
        tunnel: w315 -> [w330 _]
        tunnel: [w330 -0.35 ("Elevate 1")] -> w309
        tunnel: w313 -> [w329 _]
        tunnel: [w329 0.0 ("Reject no want")] -> w312
        frame False {
        }
        frame True {
        }
      }
      n141 = case shown="True" w310 {
        tunnel: w312 -> [w326 _]
        tunnel: [w326 -1.0 ("Reject no want")] -> w311
        tunnel: w309 -> [w325 _]
        tunnel: [w325 1.0 ("Elevate 1")] -> w308
        frame False {
        }
        frame True {
        }
      }
    }
  }
  n142 = case shown="True" w38 {
    frame False {
      n143 = call-poly <vilib>:"NT Write Value.vi"("Boolean"=FALSE, "Name"="Accept") -> ()  [unwired: 9 in, 1 out]
    }
    frame True {
      n144 = call-poly <vilib>:"NT Write Value.vi"("Boolean"=TRUE, "Name"="Accept") -> ()  [unwired: 9 in, 1 out]
    }
  }
  n145 = call <vilib>:"WPI_SolenoidRefNum Registry Get.vi"("refnum name"="Intake Solenoid") -> ("error out"=w101:errorcluster, "SolenoidDevRef"=w100:T11)  [unwired: 9 in]
  n146 = call <vilib>:"CTRE_Phoenix_MotorControl_RefNumRegistryGet.vi"("refnum name"="Elevate") -> ("error out"=w138:errorcluster, "PhoenixMotorControlDevRef"=w137:T6)  [unwired: 9 in]
  n147 = call <vilib>:"CTRE_Phoenix_MotorControl_RefNumRegistryGet.vi"("refnum name"="Reject") -> ("error out"=w140:errorcluster, "PhoenixMotorControlDevRef"=w139:T6)  [unwired: 9 in]
  n148 = call <vilib>:"CTRE_Phoenix_MotorControl_RefNumRegistryGet.vi"("refnum name"="Intake") -> ("error out"=w142:errorcluster, "PhoenixMotorControlDevRef"=w141:T6)  [unwired: 9 in]
  n149 = call-poly <vilib>:"WPI_SolenoidSet.vi"("error in (no error)"=w101, "Value"=w36, "SolenoidDevRef"=w100) -> ()  [unwired: 7 in, 2 out]
  n150 = call <vilib>:"CTRE_Phoenix_MotorControl_Set.vi"("error in (no error)"=w140, "Output"=w40, "Control Mode"=w131, "PhoenixMotorControlDevRef"=w139) -> ()  [unwired: 6 in, 2 out]
  n151 = call <vilib>:"CTRE_Phoenix_MotorControl_Set.vi"("error in (no error)"=w142, "Output"=w41, "Control Mode"=w132, "PhoenixMotorControlDevRef"=w141) -> ()  [unwired: 6 in, 2 out]
  n152 = call <vilib>:"CTRE_Phoenix_MotorControl_Set.vi"("error in (no error)"=w138, "Output"=w42, "Control Mode"=w133, "PhoenixMotorControlDevRef"=w137) -> ()  [unwired: 6 in, 2 out]
